vi "Wrap Data.vi"(7 "Start Time":timestamp, 8 "error in (no error)":errorcluster, 9 "Data in":refnum<class "Data.lvclass">, 10 "Actor in":refnum<class "Actor.lvclass">, 11 "Instrument Msg":refnum<class "Instrument Msg.lvclass">) -> (0 "error out":errorcluster, 1 "Data out":refnum<class "Data.lvclass">, 2 "Actor out":refnum<class "Actor.lvclass">)   [LabVIEW 2020, in "Instrument Handler.lvlib" / "Instrument Msg.lvclass"]
doc: "The Wrap Data VI allows the Actor and/or message to interact with the data before it is sent or published.\n\nThis implementation adds the Instrument ID if the Data is part of the Instrument Data hierarchy."
uses:
  Instrument Msg.lvclass
  PPL/HDH.Actor Framework.Core.Actor.lvlibp/1abvi3w/vi.lib/ActorFramework/Actor/Actor.lvclass
  PPL/HDH.Data.Generic.lvlibp/Data.lvclass
  Instrument Owner/Instrument Owner.lvclass
  C:/Current projects/WS/PPL/HDH.Actor Framework.Core.Actor.lvlibp/1abvi3w/vi.lib/ActorFramework/Actor/Actor.lvclass
  Data/Instrument Data/Instrument Data.lvclass
  C:/Current projects/WS/PPL/HDH.Data.Generic.lvlibp/Data.lvclass
  Instrument Owner/Instrument Owner.lvclass/Instrument Owner.ctl
  Data/Instrument Data/Instrument Data.lvclass/Instrument Data.ctl
  PPL/HDH.Actor Framework.Core.Publisher.lvlibp/Messages/Timed Msg/Timed Msg.lvclass
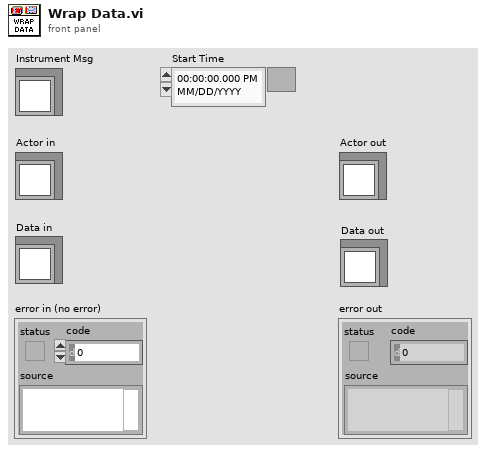
[diagram p1: front panel]
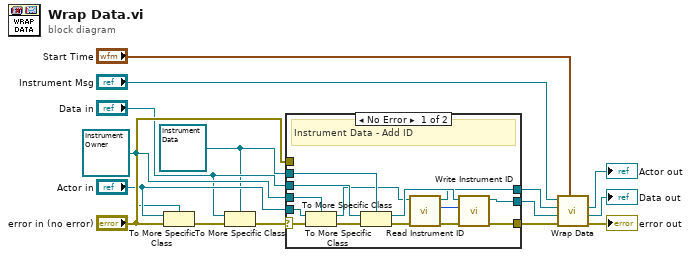
[diagram p0: block diagram]
diagram:
  w1 = refnum<class "Instrument Data.lvclass"> refnum ("Instrument Handler.lvlib:Instrument Data.lvclass")
  w5 = refnum<class "Instrument Owner.lvclass"> refnum ("Instrument Handler.lvlib:Instrument Owner.lvclass")
  n1 = To More Specific Class(target class=w5, reference="Actor in", error in="error in (no error)") -> (error out=w3:errorcluster)  [unwired: 1 out]
  n2 = To More Specific Class(target class=w1, reference="Data in", error in=w3) -> (error out=w2:errorcluster)  [unwired: 1 out]
  n3 = case "Write instrument ID to data" shown="No Error" w2 {
    selector: w2 -> [w29 _]
    tunnel: [w20 w32] -> w10
    tunnel: "Actor in" -> [w16 w32]
    tunnel: [w23 w31] -> w8
    tunnel: "error in (no error)" -> [_ w31]
    tunnel: [w22 w30] -> w7
    tunnel: "Data in" -> [w25 w30]
    tunnel: w5 -> [w28 _]
    tunnel: w1 -> [w26 _]
    frame No Error {
      # "Instrument Data - Add ID"
      n4 = To More Specific Class(target class=w28, reference=w16, error in=w29) -> (specific class reference=w21:refnum<class "Instrument Owner.lvclass">, error out=w27:errorcluster)
      n5 = To More Specific Class(target class=w26, reference=w25, error in=w27) -> (specific class reference=w24:refnum<class "Instrument Data.lvclass">, error out=w18:errorcluster)
      n6 = call "Read Instrument ID.vi"("error in (no error)"=w18, "Instrument Owner in"=w21) -> ("error out"=w17:errorcluster, "Instrument ID out"=w19:u32, "Instrument Owner out"=w20:refnum<class "Instrument Owner.lvclass">)  [unwired: 7 in]
      n7 = call "Write Instrument ID.vi"("error in (no error)"=w17, "Instrument ID"=w19, "Instrument Data in"=w24) -> ("error out"=w23:errorcluster, "Instrument Data out"=w22:refnum<class "Instrument Data.lvclass">)  [unwired: 7 in]
    }
    frame Error {
      # "Not Instrument Data - Skip"
    }
  }
  n8 = call-parent "Wrap Data.vi"("Start Time"="Start Time", "error in (no error)"=w8, "Data in"=w7, "Actor in"=w10, "Timed Msg"="Instrument Msg") -> ("error out"=→"error out":errorcluster, "Data out"=→"Data out":refnum<class "Data.lvclass">, "Actor out"=→"Actor out":refnum<class "Actor.lvclass">)  [unwired: 4 in]
